vi "Grab Hatch Panel in Auto.vi"   [LabVIEW 2018]
uses:
  SubSystems/Hatch Panel Intake/Hatch Panel Intake Global.vi
  SubSystems/Cargo Intake/Cargo Intake Global.vi
  SubSystems/Lift/Lift Global.vi
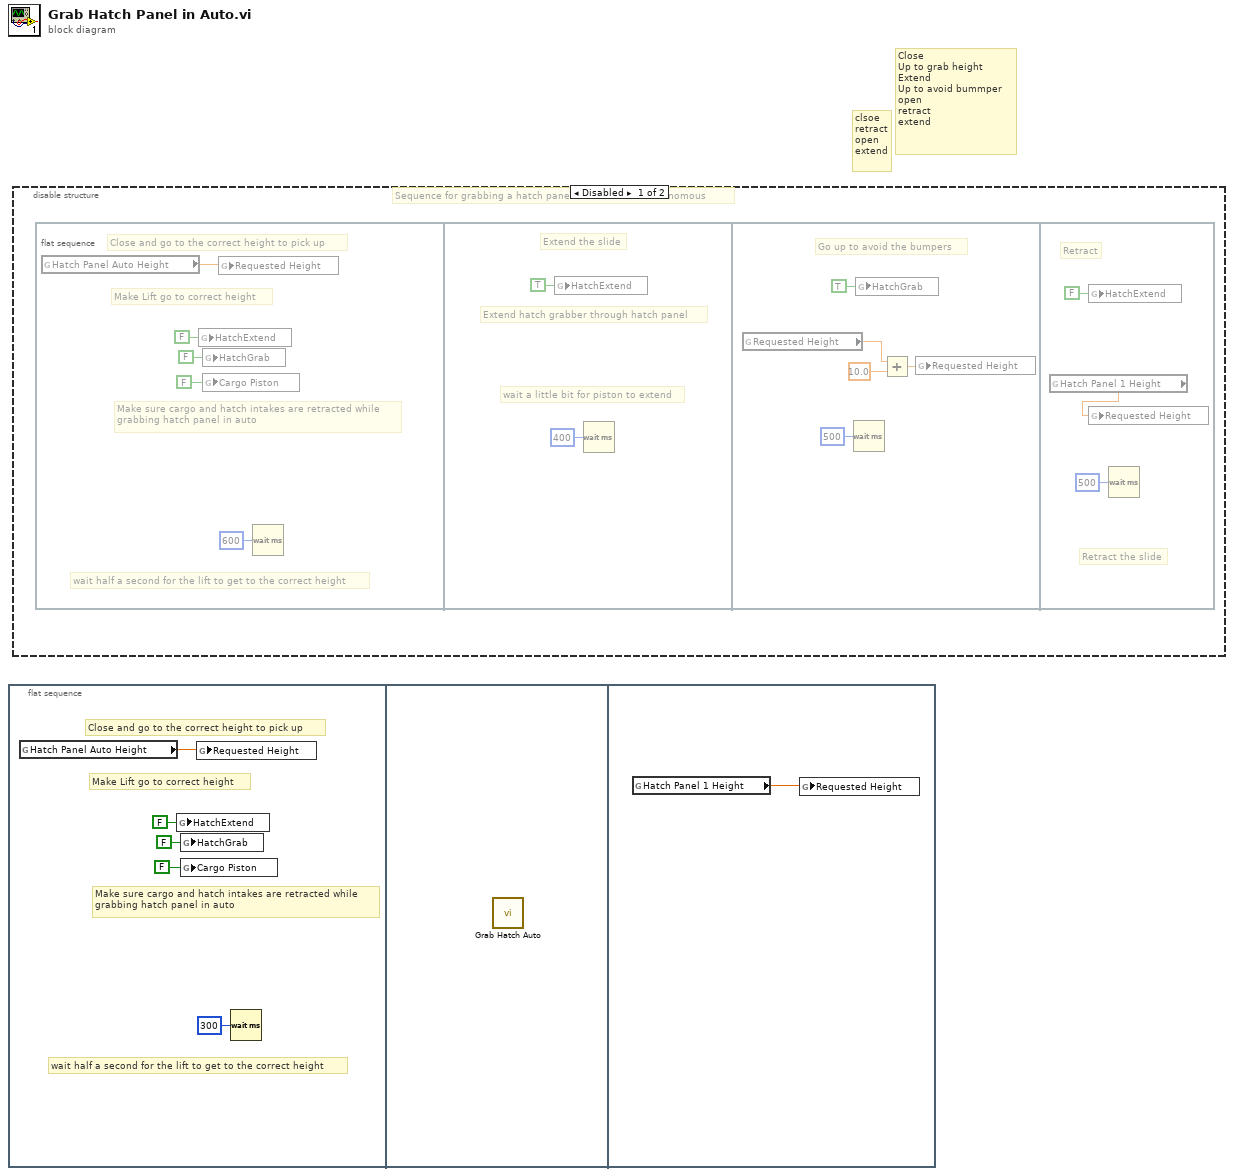
[diagram p0: block diagram]
diagram:
  # "clsoe\nretract\nopen\nextend"
  # "Close\nUp to grab height\nExtend\nUp to avoid bummper\nopen\nretract\nextend"
  n1 = flat-sequence {
    frame #0 {
      # "Close and go to the correct height to pick up"
      # "Make sure cargo and hatch intakes are retracted while\ngrabbing hatch panel in auto"
      # "wait half a second for the lift to get to the correct height"
      # "Make Lift go to correct height"
      n2 = global read "Lift Global.vi" "Hatch Panel Auto Height"() -> (w5:dbl)
      n3 = global write "Hatch Panel Intake Global.vi" "HatchExtend"(FALSE ("HatchExtend")) -> ()
      n4 = global write "Hatch Panel Intake Global.vi" "HatchGrab"(FALSE ("HatchGrab")) -> ()
      n5 = global write "Cargo Intake Global.vi" "Cargo Piston"(FALSE ("Cargo Piston")) -> ()
      n6 = global write "Lift Global.vi" "Requested Height"(w5) -> ()
      n7 = Wait (ms)(milliseconds to wait=u32 300) -> ()  [unwired: 1 out]
    }
    frame #1 {
      n8 = call "Grab Hatch Auto.vi"() -> ()  [unwired: 12 in]
    }
    frame #2 {
      n9 = global read "Lift Global.vi" "Hatch Panel 1 Height"() -> (w6:dbl)
      n10 = global write "Lift Global.vi" "Requested Height"(w6) -> ()
    }
  }
  n11 = disable-structure shown="Disabled" {
    frame Disabled {
      # "Sequence for grabbing a hatch panel at the start of autonomous"
      n12 = flat-sequence {
        frame #0 {
          # "Close and go to the correct height to pick up"
          # "Make sure cargo and hatch intakes are retracted while\ngrabbing hatch panel in auto"
          # "wait half a second for the lift to get to the correct height"
          # "Make Lift go to correct height"
          n13 = global read "Lift Global.vi" "Hatch Panel Auto Height"() -> (w11:dbl)
          n14 = global write "Hatch Panel Intake Global.vi" "HatchExtend"(FALSE ("HatchExtend")) -> ()
          n15 = global write "Hatch Panel Intake Global.vi" "HatchGrab"(FALSE ("HatchGrab")) -> ()
          n16 = global write "Cargo Intake Global.vi" "Cargo Piston"(FALSE ("Cargo Piston")) -> ()
          n17 = global write "Lift Global.vi" "Requested Height"(w11) -> ()
          n18 = Wait (ms)(milliseconds to wait=u32 600) -> ()  [unwired: 1 out]
        }
        frame #1 {
          # "Extend the slide"
          # "wait a little bit for piston to extend"
          # "Extend hatch grabber through hatch panel"
          n19 = global write "Hatch Panel Intake Global.vi" "HatchExtend"(TRUE ("HatchExtend")) -> ()
          n20 = Wait (ms)(milliseconds to wait=u32 400) -> ()  [unwired: 1 out]
        }
        frame #2 {
          # "Go up to avoid the bumpers"
          n21 = global read "Lift Global.vi" "Requested Height"() -> (w16:dbl)
          n22 = Wait (ms)(milliseconds to wait=u32 500) -> ()  [unwired: 1 out]
          n23 = global write "Hatch Panel Intake Global.vi" "HatchGrab"(TRUE ("HatchGrab")) -> ()
          n24 = Add(x=w16, y=10.0) -> (x+y=w17:dbl)
          n25 = global write "Lift Global.vi" "Requested Height"(w17) -> ()
        }
        frame #3 {
          # "Retract"
          # "Retract the slide"
          n26 = global read "Lift Global.vi" "Hatch Panel 1 Height"() -> (w19:dbl)
          n27 = global write "Hatch Panel Intake Global.vi" "HatchExtend"(FALSE ("HatchExtend")) -> ()
          n28 = global write "Lift Global.vi" "Requested Height"(w19) -> ()
          n29 = Wait (ms)(milliseconds to wait=u32 500) -> ()  [unwired: 1 out]
        }
      }
    }
    frame Enabled {
    }
  }
